vi "detectorTrama.vi"(0 "VISA resource name":refnum<visa-resource-name>, 1 "error in (no error)":errorcluster) -> (2 "VISA resource name 2":refnum<visa-resource-name>, 3 "Numeric":i32, 4 "error in (no error) 2":errorcluster)   [LabVIEW 2011]
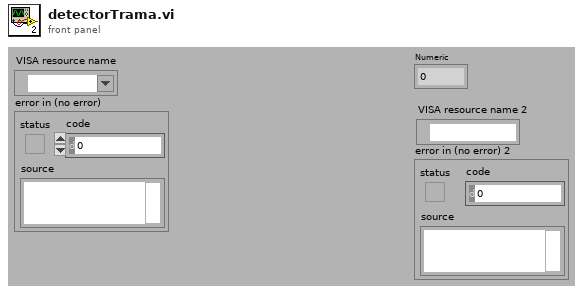
[diagram p1: front panel]
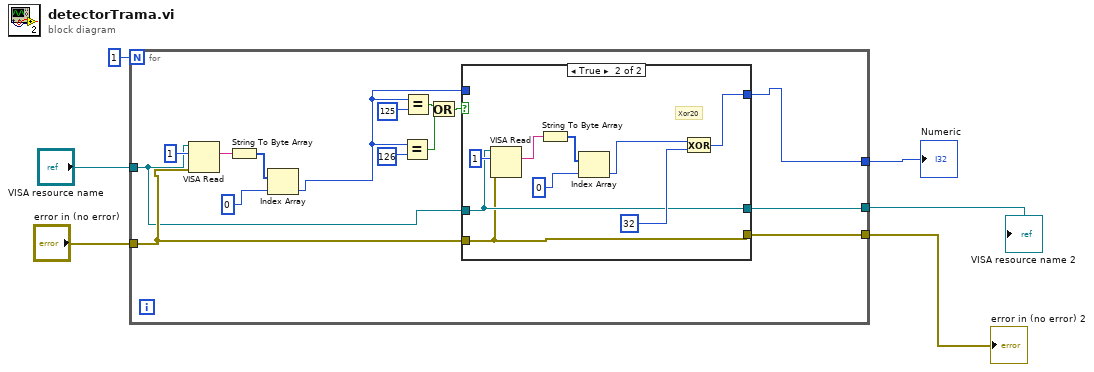
[diagram p0: block diagram]
diagram:
  n1 = for {
    N: 1 -> [_]
    tunnel: "error in (no error)" -> [w12]
    tunnel: "VISA resource name" -> [w11]
    tunnel: [w10] -> w2
    tunnel: [w9] -> w4
    tunnel: [w8] -> w3
    n2 = VISA Read(VISA resource name=w11, byte count=u32 1, error in (no error)=w12) -> (read buffer=w15:string)  [unwired: 3 out]
    n3 = String To Byte Array(string=w15) -> (unsigned byte array=w13:u8[])
    n4 = Index Array(array=w13, index=0) -> (element=w7:u8)
    n5 = Equal?(x=w7, y=u16 126) -> (x = y?=w19:bool)
    n6 = Equal?(x=w7, y=u16 125) -> (x = y?=w18:bool)
    n7 = Or(x=w18, y=w19) -> (x .or. y?=w17:bool)
    n8 = case shown="True" w17 {
      tunnel: w7 -> [w24 _]
      tunnel: [w24 w32] -> w10
      tunnel: w11 -> [w23 w26]
      tunnel: w12 -> [w22 w25]
      tunnel: [w23 w26] -> w9
      tunnel: [w22 w25] -> w8
      frame False {
      }
      frame True {
        # "Xor20"
        n9 = VISA Read(VISA resource name=w26, byte count=u32 1, error in (no error)=w25) -> (read buffer=w31:string)  [unwired: 3 out]
        n10 = String To Byte Array(string=w31) -> (unsigned byte array=w29:u8[])
        n11 = Index Array(array=w29, index=0) -> (element=w28:u8)
        n12 = Exclusive Or(1:32 ("y"), 2:w28) -> (0:w32:i32)
      }
    }
  }
  "VISA resource name 2" <- w4
  "error in (no error) 2" <- w3
  "Numeric" <- w2
